vi "kuirs_双相机_1.vi"() -> ()   [LabVIEW 2019]
uses:
  <vilib>/userdefined/High Color/IMAQdx.ctl
  <vilib>/vision/driver/NI_Vision_Acquisition_Software.lvlib
panel:
  in  "Session In":T1
  out "Image":T2(plugin-control)
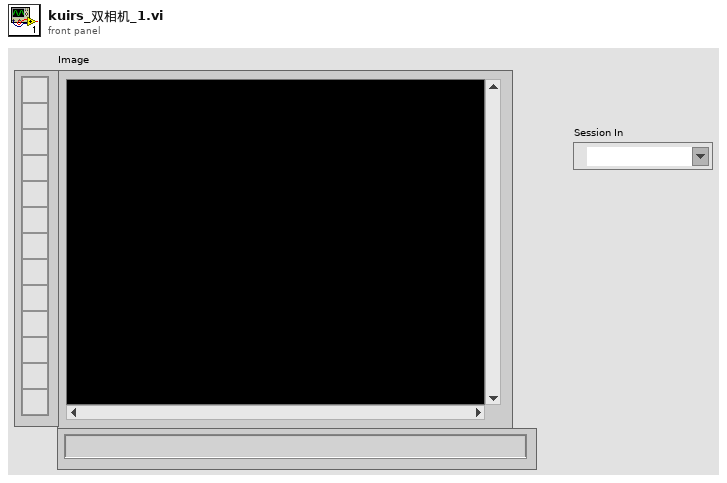
[diagram p1: front panel]
types:
  T1 = typedef "IMAQdx.ctl" = refnum<k21>
  T2 = typedef "IMAQ Image.ctl" = refnum<image>
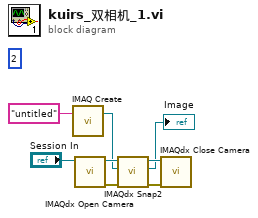
[diagram p0: block diagram]
diagram:
  (unwired) 2
  n1 = call "IMAQ Create"("Image Name"="untitled") -> ("New Image"=w6:T2)  [unwired: 4 in, 1 out]
  n2 = call <vilib>:"IMAQdx Open Camera.vi"("Session In"="Session In") -> ("error out"=w3:errorcluster, "Session Out"=w8:T1)  [unwired: 9 in]
  n3 = call <vilib>:"IMAQdx Snap2.vi"("error in"=w3, "Image In"=w6, "Session In"=w8) -> ("error out"=w4:errorcluster, "Image Out"=→"Image":T2, "Session Out"=w5:T1)  [unwired: 6 in]
  n4 = call <vilib>:"IMAQdx Close Camera.vi"("error in"=w4, "Session In"=w5) -> ()  [unwired: 9 in, 1 out]
